vi "transparent array cluster.vi"() -> ()   [LabVIEW 2020]
uses:
  Controls/UI-Digital Pin.ctl
panel:
  in  "Cluster":T1 {"Pin Value" format="%#_g V"}
  in  "Cluster (transparent)":cluster{}
  in  "Array Of Cluster with 2 Strings":T2(array[cluster])=[{"String Indicator (transparent)"="cd", "String Indicator (transparent) 2"="ab"}, {"String Indicator (transparent)"="ab", "String Indicator (transparent) 2"="fas"}]
  in  "String Indicator (transparent)":string
  in  "Array (transparent":void[](array[numeric])
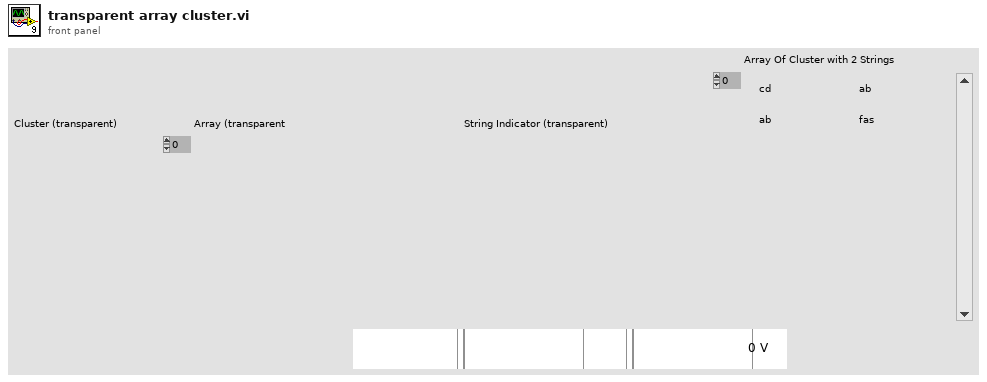
[diagram p1: front panel]
types:
  T1 = typedef "UI-Digital Pin.ctl" = cluster{"IO Direction":u16, "Pin Direction":string, "DO Value":u16, "Pin Value":dbl, "Pin Index":string, "Pin Mode":string}
  T2 = cluster{"String Indicator (transparent)":string, "String Indicator (transparent) 2":string}[]
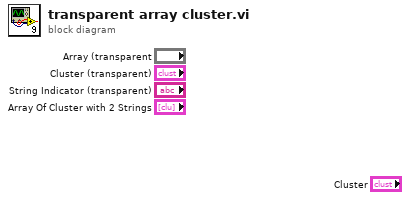
[diagram p0: block diagram]
diagram:
